vi "random alphas.vi"() -> ()   [LabVIEW 2009]
panel:
  out "string":string
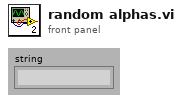
[diagram p1: front panel]
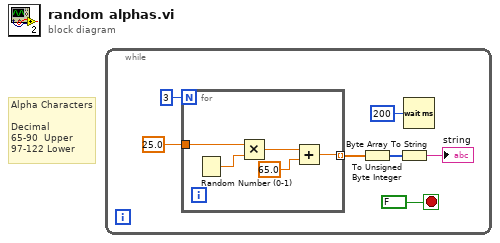
[diagram p0: block diagram]
diagram:
  # "Alpha Characters\n\nDecimal \n65-90  Upper\n97-122 Lower"
  n1 = while {
    stop <- FALSE stop-if-true
    n2 = for {
      N: 3 -> [_]
      tunnel: 25.0 -> [w9]
      tunnel: [w8] -> w5 mode=indexing
      n3 = Random Number (0-1)() -> (number: 0 to 1=w12:dbl)
      n4 = Multiply(x=w9, y=w12) -> (x*y=w10:dbl)
      n5 = Add(x=w10, y=65.0) -> (x+y=w8:dbl)
    }
    n6 = To Unsigned Byte Integer(number=w5) -> (unsigned 8bit integer=w3:u8[])
    n7 = Byte Array To String(unsigned byte array=w3) -> (string=→"string":string)
    n8 = Wait (ms)(milliseconds to wait=u32 200) -> ()  [unwired: 1 out]
  }
